vi "hopper inf log.vi"   [LabVIEW 2014]
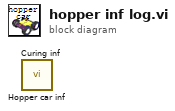
[diagram p0: block diagram]
diagram:
  n1 = call "Hopper car inf.vi"() -> ()  [unwired: 10 in, 2 out]
  n2 = call "Curing inf.vi"() -> ()  [unwired: 10 in, 2 out]
